vi "espaceSpecCharacters.vi"(8 "error in":errorcluster, 11 "StringIN":string) -> (0 "error out":errorcluster, 3 "StringOUT":string)   [LabVIEW 2011, in "JSON.lvlib"]
uses:
  JSON.lvlib
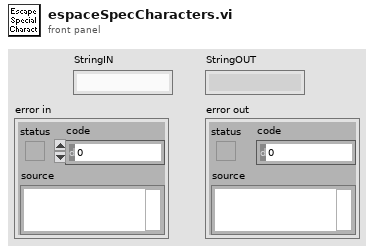
[diagram p1: front panel]
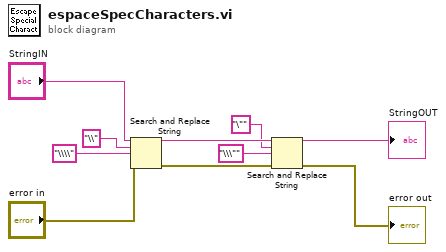
[diagram p0: block diagram]
diagram:
  n1 = Search and Replace String(input string="StringIN", search string="\\", replace string="\\\\" ("replace string (\"\")"), error in="error in") -> (result string=w8:string, error out=w7:errorcluster)  [unwired: 4 in, 2 out]
  n2 = Search and Replace String(input string=w8, search string="\"", replace string="\\\"" ("replace string (\"\")"), error in=w7) -> (result string=→"StringOUT":string, error out=→"error out":errorcluster)  [unwired: 4 in, 2 out]
